vi "Ic_Create_CGH.vi"(0 "2D array in":u8[][](array[numeric]), 1 "Repetition Number":u32, 2 "progressBarOFF_0_ON_1":u8, 3 "error in (no error)":errorcluster) -> (7 "2D array out":u8[][](array[numeric]), 10 "error out":errorcluster)   [LabVIEW 2016]
uses:
  LabVIEW2018/Image_Control.dll
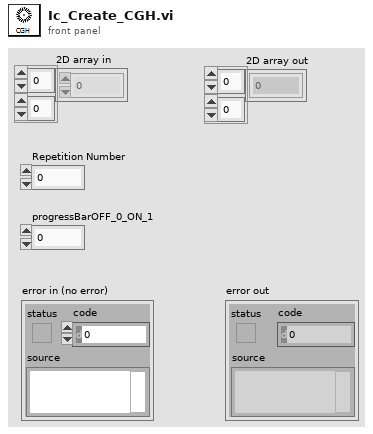
[diagram p1: front panel]
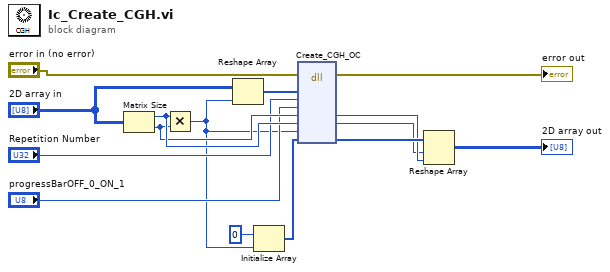
[diagram p0: block diagram]
diagram:
  n1 = Matrix Size(0:"2D array in") -> (1:w10:i32, 2:w9:i32)
  n2 = Multiply(x=w10, y=w9) -> (x*y=w6:i32)
  n3 = Reshape Array("2D array in", w6) -> (w11:u8[])
  n4 = Initialize Array(u8 0 ("要素"), w6) -> (w5:u8[])
  n5 = dll-call lib="C:/Users/hs5921/Desktop/LabVIEW2018/Image_Control.dll" fn="Create_CGH_OC"(error in="error in (no error)", "1DArrayIn"=w11, "RepetitionNumber"="Repetition Number", "progressBarOFF_0_ON_1"="progressBarOFF_0_ON_1", "X_pixel_target"=w9, "Y_pixel_target"=w10, "targetDataSize"=w6, "1DArrayOut"=w5) -> (error out=→"error out":errorcluster, "X_pixel_target"=w3:i32, "Y_pixel_target"=w2:i32, "1DArrayOut"=w4:u8[])  [unwired: 7 in, 1 out]
  n6 = Reshape Array(w4, w2, w3) -> (→"2D array out":u8[][])
